vi "polling read.vi"() -> ()   [LabVIEW 2020]
uses:
  LabVIEW-MIDI-XPLAT/LabVIEW-MIDI-XPLAT.lvclass
panel:
  out "return":i32
  out "Return 2":i32
  out "Return":i32
  in  "Stop":bool
  out "buffer":u8[](array[numeric])
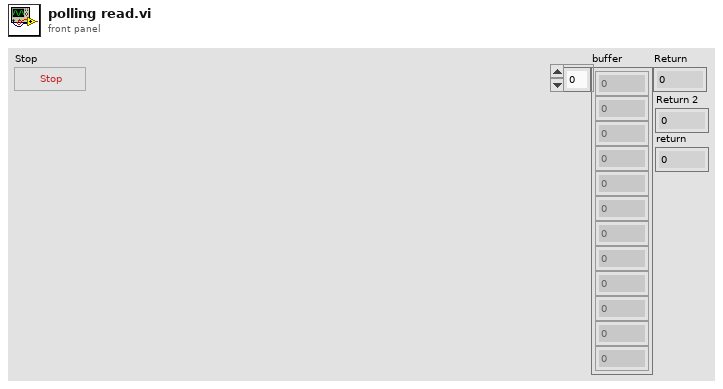
[diagram p1: front panel]
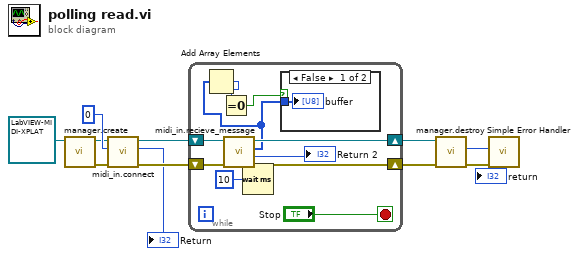
[diagram p0: block diagram]
diagram:
  n1 = call "manager.create.vi"("LabVIEW-MIDI-XPLAT in"=refnum<class "LabVIEW-MIDI-XPLAT.lvclass"> refnum) -> ("error out"=w9:errorcluster, "LabVIEW-MIDI-XPLAT out"=w10:refnum<class "LabVIEW-MIDI-XPLAT.lvclass">)  [unwired: 9 in]
  n2 = call "midi_in.connect.vi"("error in (no error)"=w9, "device_index"=0, "LabVIEW-MIDI-XPLAT in"=w10) -> ("error out"=w7:errorcluster, "Return"=→"Return":i32, "LabVIEW-MIDI-XPLAT out"=w8:refnum<class "LabVIEW-MIDI-XPLAT.lvclass">)  [unwired: 6 in]
  n3 = while {
    shift-right: [w19] -> w6
    shift-left: w8 -> [w21]
    shift-right: [w18] -> w5
    shift-left: w7 -> [w20]
    stop <- "Stop" stop-if-true
    n4 = call "midi_in.recieve_message.vi"("error in (no error)"=w20, "LabVIEW-MIDI-XPLAT in"=w21) -> ("error out"=w18:errorcluster, "Return"=→"Return 2":i32, "buffer"=w14:u8[], "LabVIEW-MIDI-XPLAT out"=w19:refnum<class "LabVIEW-MIDI-XPLAT.lvclass">)  [unwired: 6 in]
    n5 = Add Array Elements(numeric array=w14) -> (sum=w13:u8)
    n6 = Equal To 0?(x=w13) -> (x = 0?=w15:bool)
    n7 = Wait (ms)(milliseconds to wait=u32 10) -> ()  [unwired: 1 out]
    n8 = case shown="False" w15 {
      tunnel: w14 -> [w22 _]
      frame False {
        "buffer" <- w22
      }
      frame True {
      }
    }
  }
  n9 = call "manager.destroy.vi"("error in (no error)"=w5, "LabVIEW-MIDI-XPLAT in"=w6) -> ("error out"=w3:errorcluster, "return"=→"return":i32)  [unwired: 7 in, 1 out]
  n10 = call <vilib>:"Simple Error Handler.vi"("error in (no error)"=w3) -> ()  [unwired: 4 in, 5 out]
